vi "Create_AO_Signal4Z.vi"(8 "error in":errorcluster, 10 "AO Amplitude":dbl(slide) min=0.0 max=100.0 step=1.0 scale=0.0..100.0, 11 "ON / OFF":bool=TRUE) -> (0 "error out":errorcluster, 3 "WF":dbl[](array[numeric]))   [LabVIEW 2025]
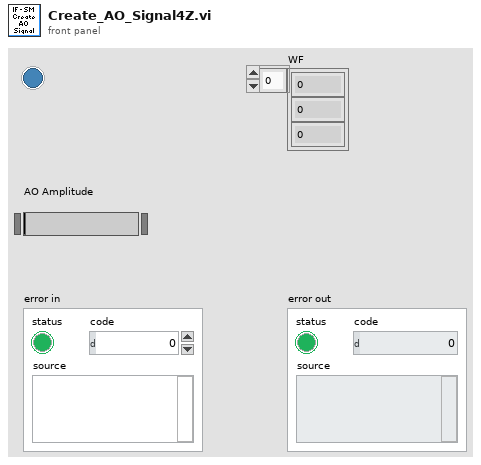
[diagram p1: front panel]
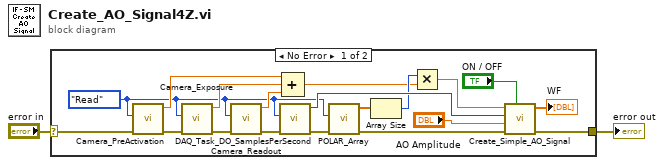
[diagram p0: block diagram]
diagram:
  n1 = case shown="No Error" "error in" {
    selector: "error in" -> [w21 w22]
    tunnel: [w12 w22] -> w1
    frame No Error {
      w7 = enum16{"Write", "Read"}."Read" ("Action")
      n2 = call "Camera_PreActivation.vi"("error in"=w21, "Action"=w7) -> ("error out"=w20:errorcluster, "Camera_PreActivation"=w16:dbl)  [unwired: 8 in]
      n3 = call "Camera_Exposure.vi"("error in"=w20, "Action"=w7) -> ("error out"=w19:errorcluster, "Exposure (s)"=w15:dbl)  [unwired: 8 in]
      n4 = call "Camera_Readout.vi"("error in"=w19, "Action"=w7) -> ("error out"=w18:errorcluster, "Camera_Readout"=w10:dbl)  [unwired: 8 in]
      n5 = call "DAQ_Task_DO_SamplesPerSecond.vi"("error in"=w18, "Action"=w7) -> ("error out"=w9:errorcluster, "DO_Task_SamplesPerSec"=w13:u32)  [unwired: 8 in]
      n6 = Compound Arithmetic op=ADD(w16, w15, w10) -> (w4:dbl)
      n7 = call "POLAR_Array.vi"("error in"=w9, "Action"=w7) -> ("error out"=w8:errorcluster, "Pockels_Array"=w6:dbl[])  [unwired: 8 in]
      n8 = Array Size(array=w6) -> (size(s)=w5:i32)
      n9 = Multiply(x=w5, y=w4) -> (x*y=w3:dbl)
      n10 = call "Create_Simple_AO_Signal.vi"("On/OFF"="ON / OFF", "error in"=w8, "Amplitude"="AO Amplitude", "Samples / s (10000)"=w13, "Time (s)"=w3) -> ("error out"=w12:errorcluster, "Signal"=→"WF":dbl[])  [unwired: 5 in]
    }
    frame Error {
    }
  }
  "error out" <- w1
